vi "CONTROL LIFT ARM.vi"(10 "LIFT ARM refname":string="INTAKE LIFT", 11 "LIFT DRIVE refname":string="INTAKE DRIVE") -> ()   [LabVIEW 2020]
uses:
  <vilib>/Rock Robotics/WPI/ThirdParty/Phoenix-LabVIEW/Motor Controller/Controls/CTRE_Phoenix_MotorControl_ControlMode.ctl
  <vilib>/Rock Robotics/Network Tables/NT Read Boolean.vi
  Robot Global Data.vi
  <vilib>/Rock Robotics/Network Tables/NT Write Boolean.vi
panel:
  out "Sensor Position RETRACT":dbl
  out "TARGET RETRACT":dbl
  out "TARGET EXTEND":dbl
  out "Sensor Position EXTEND":dbl
  in  "degrees overtravel":dbl=5.0 format="%#_13g"
  out "LOOP ITERATION LIMIT?":bool
  out "THRESHOLD?":bool
  out "AND nots":bool[](array[boolean])=[TRUE, FALSE, FALSE, FALSE]
  out "NOT XOR":bool[](array[boolean])=[TRUE, FALSE, FALSE, TRUE]
  out "Not AND":bool[](array[boolean])=[TRUE, TRUE, TRUE, FALSE]
  out "AND?":bool[](array[boolean])=[FALSE, FALSE, FALSE, TRUE]
  in  "POSSIBILITIES":cluster{"EXTEND":bool, "RETRACTED":bool}[](array[cluster])=[{"EXTEND"=FALSE, "RETRACTED"=FALSE}, {"EXTEND"=TRUE, "RETRACTED"=FALSE}, {"EXTEND"=FALSE, "RETRACTED"=TRUE}, {"EXTEND"=TRUE, "RETRACTED"=TRUE}]
  out "IS RETRACTED?":bool
  out "SHOULD BE EXTENDED?":bool
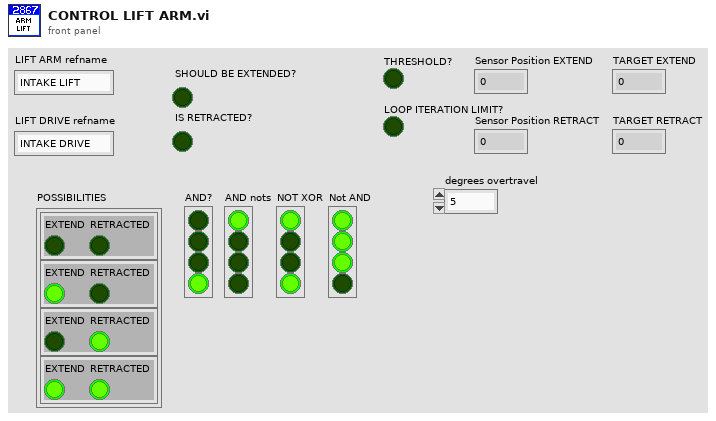
[diagram p1: front panel]
types:
  T1 = cluster{"planetary gear ratio:1":i32, "GEAR TEETH on planetary":i32, "GEAR TEETH on lift arm":i32, "convert motor revs to lift degrees":dbl, "MIN (deg)":dbl, "MAX (deg)":dbl, "roller speed%":dbl, "tip over (deg)":dbl, "lift speed% EXTEND":dbl, "lift speed% RETRACT":dbl}
  T2 = typedef "WPI_MotorControlDeviceRef.ctl" = cluster{"DeviceStatus":errorcluster, "Type":T3, "PWM":cluster{"PWM Channel":T4, "DeadBand":T5}, "CAN":cluster{"Device Number":u8, "SetOutput VI Ref":variant, "GetOutput VI Ref":variant, "Enable VI Ref":variant, "Disable VI Ref":variant, "Data":variant}, "Invert":bool, "DIO PWM":cluster{"PWM \"Enable\" Channel":T4, "DIOChannel":T6, "PWM Rate":dbl}}
  T3 = typedef "WPI_MotorControlType.ctl" = enum16{"PWM", "CAN", "DIO PWM"}
  T4 = typedef "FPGA_DIOPWMChannel.ctl" = enum8{"PWM 0", "PWM 1", "PWM 2", "PWM 3", "PWM 4", "PWM 5", "PWM 6", "PWM 7", "PWM 8", "PWM 9", "PWM MXP 0", "PWM MXP 1", "PWM MXP 2", "PWM MXP 3", "PWM MXP 4", "PWM MXP 5", "PWM MXP 6", "PWM MXP 7", "PWM MXP 8", "PWM MXP 9", "Invalid"}
  T5 = typedef "WPI_PWMDeadband.ctl" = cluster{"Name":string, "maxPositivePwm":i32, "minPositivePwm":i32, "centerPwm":i32, "maxNegativePwm":i32, "minNegativePwm":i32, "angularRange":u16}
  T6 = typedef "FPGA_DIOChannel.ctl" = enum8{"DIO 0", "DIO 1", "DIO 2", "DIO 3", "DIO 4", "DIO 5", "DIO 6", "DIO 7", "DIO 8", "DIO 9", "DIO MXP 0", "DIO MXP 1", "DIO MXP 2", "DIO MXP 3", "DIO MXP 4", "DIO MXP 5", "DIO MXP 6", "DIO MXP 7", "DIO MXP 8", "DIO MXP 9", "DIO MXP 10", "DIO MXP 11", "DIO MXP 12", "DIO MXP 13", "DIO MXP 14", "DIO MXP 15", "SPI Port CS1", "SPI Port CS2", "SPI Port CS3", "SPI Port MISO", "SPI Port MOSI", "Invalid"}
  T7 = typedef "CTRE_Phoenix_MotorControl_ControlMode.ctl" = u16
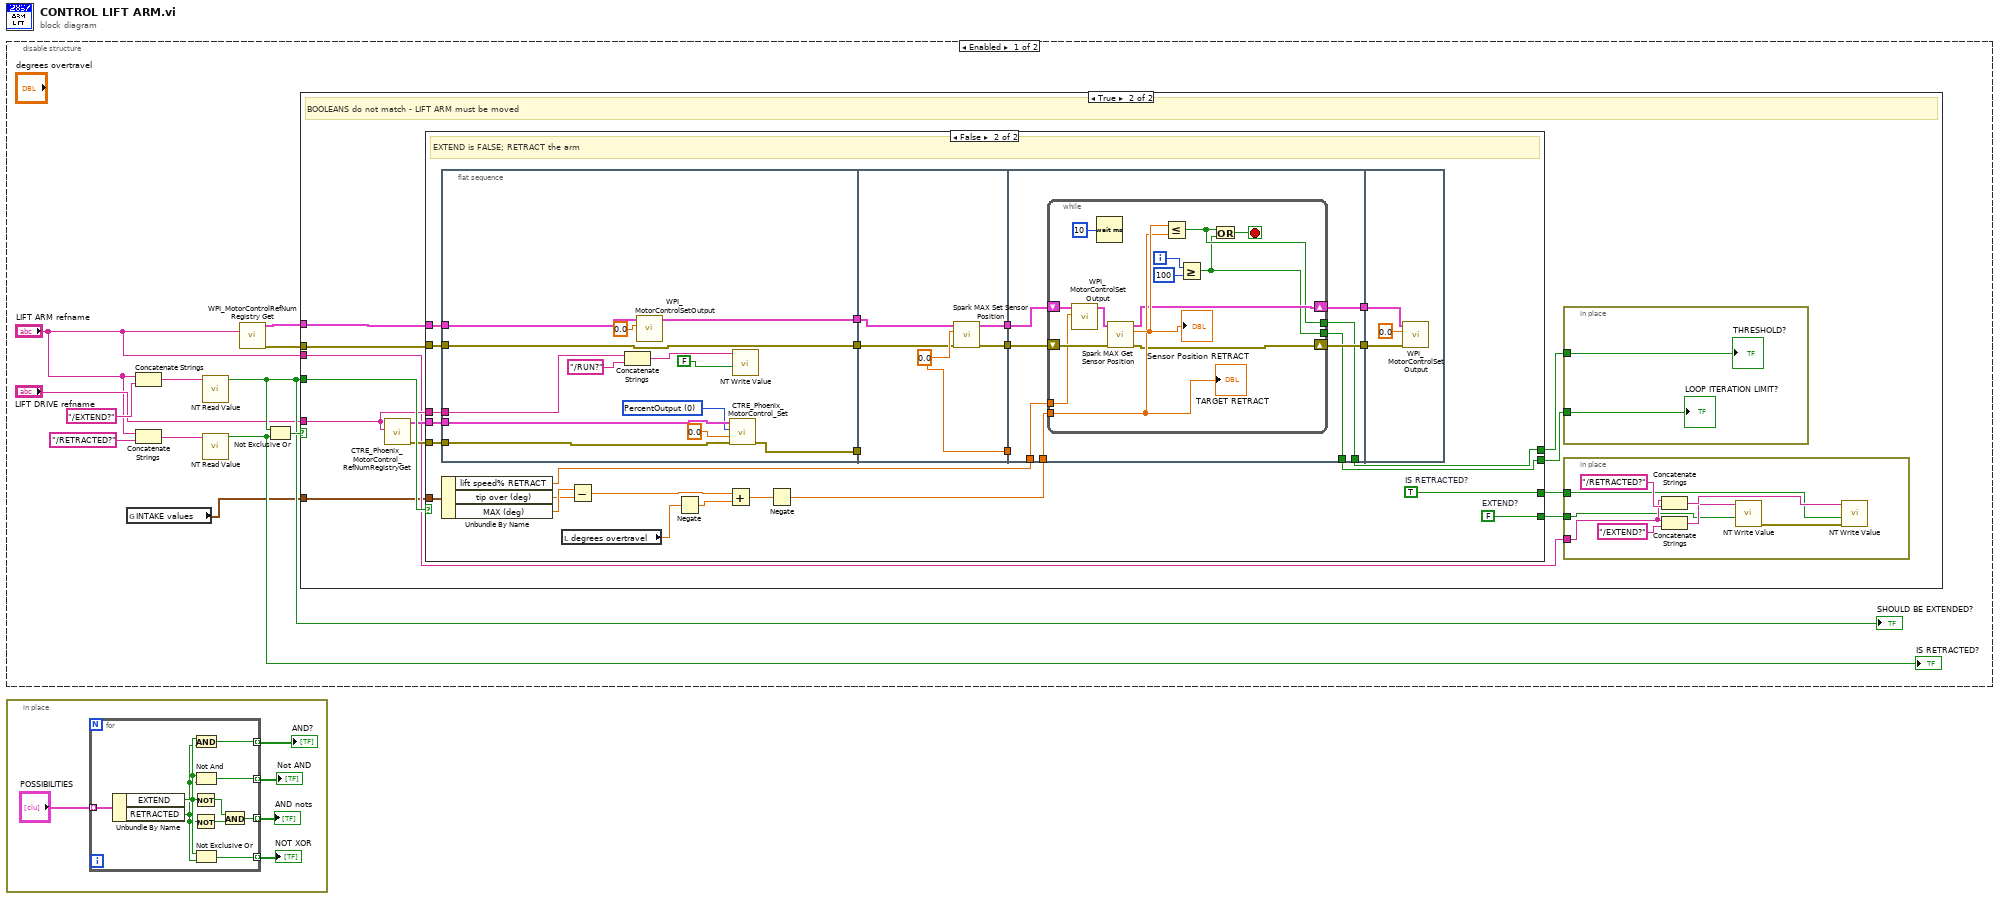
[diagram p0: block diagram]
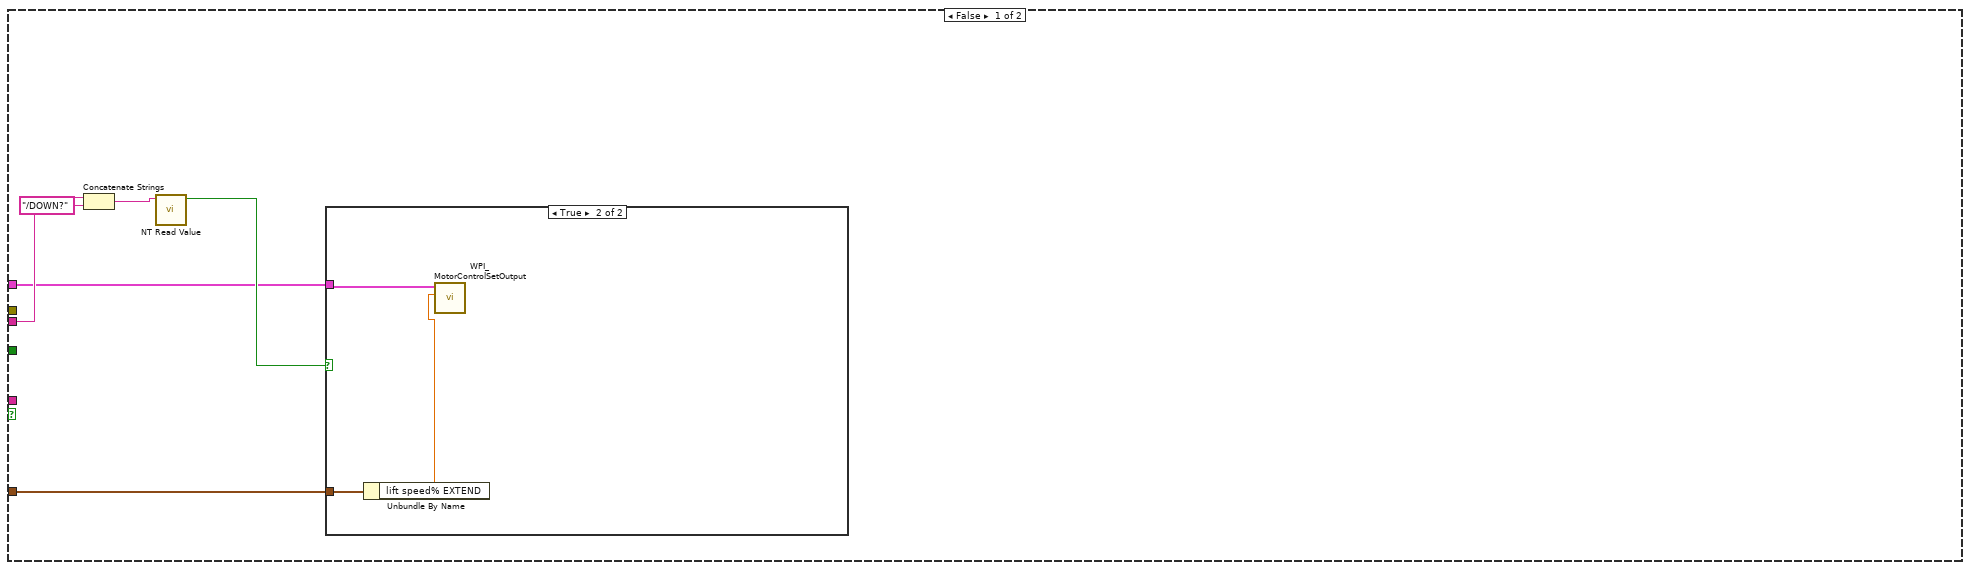
[diagram p2: hidden frame]
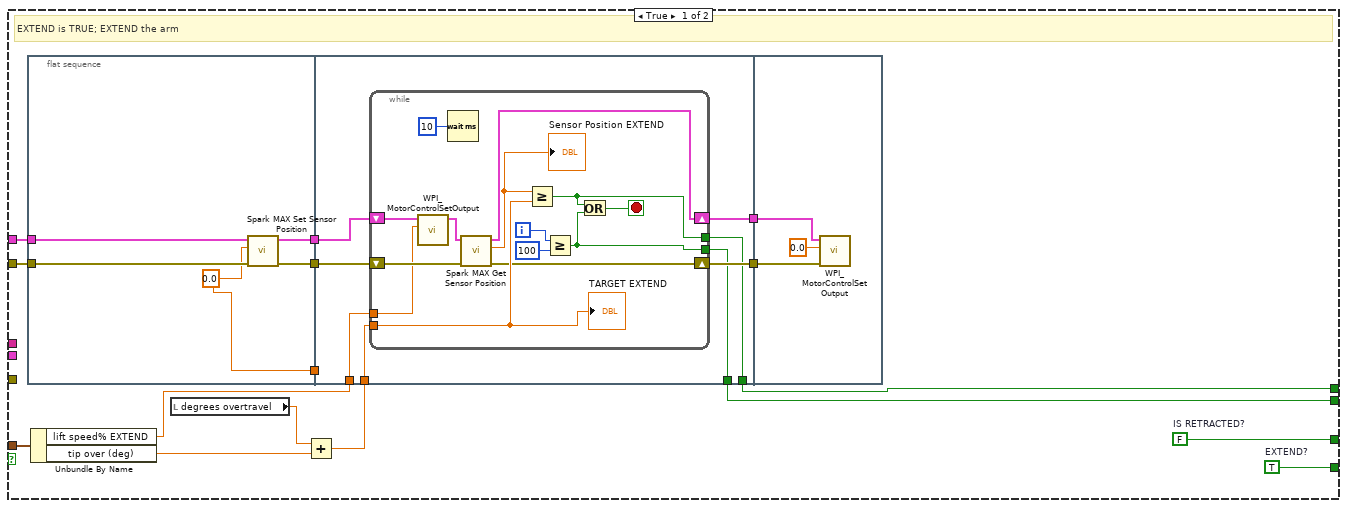
[diagram p4: hidden frame]
diagram:
  n1 = disable-structure shown="Enabled" {
    frame Enabled {
      n2 = global read "Robot Global Data.vi" "INTAKE values"() -> (w1:T1)
      n3 = Concatenate Strings("LIFT ARM refname", "/EXTEND?" ("string")) -> (w5:string)
      n4 = Concatenate Strings("LIFT ARM refname", "/RETRACTED?" ("string")) -> (w10:string)
      n5 = call-poly <vilib>:"NT Read Value.vi"("Name"=w5) -> ("Boolean"=w7:bool)  [unwired: 9 in, 1 out]
      "SHOULD BE EXTENDED?" <- w7
      n6 = call-poly <vilib>:"NT Read Value.vi"("Name"=w10) -> ("Boolean"=w9:bool)  [unwired: 9 in, 1 out]
      "IS RETRACTED?" <- w9
      n7 = call <vilib>:"WPI_MotorControlRefNum Registry Get.vi"("refnum name"="LIFT ARM refname") -> ("error out"=w3:errorcluster, "MotorControlDevRef"=w2:T2)  [unwired: 9 in]
      n8 = Not Exclusive Or(1:w9, 2:w7) -> (0:w8:bool)
      n9 = case shown="True" w8 {
        tunnel: w7 -> [_ w33]
        tunnel: "LIFT DRIVE refname" -> [_ w26]
        tunnel: "LIFT ARM refname" -> [w18 w25]
        tunnel: w3 -> [_ w24]
        tunnel: w2 -> [w14 w23]
        tunnel: w1 -> [w13 w22]
        frame False {
          n10 = Concatenate Strings(w18, "/DOWN?" ("string")) -> (w17:string)
          n11 = call-poly <vilib>:"NT Read Value.vi"("Name"=w17) -> ("Boolean"=w15:bool)  [unwired: 9 in, 1 out]
          n12 = case shown="True" w15 {
            tunnel: w14 -> [_ w20]
            tunnel: w13 -> [_ w21]
            frame False {
            }
            frame True {
              n13 = Unbundle By Name(w21) -> ("lift speed% EXTEND"=w19:dbl)
              n14 = call <vilib>:"WPI_MotorControlSetOutput.vi"("Output"=w19, "MotorControlDevRef"=w20) -> ()  [unwired: 7 in, 3 out]
            }
          }
        }
        frame True {
          # "BOOLEANS do not match - LIFT ARM must be moved"
          n15 = call <vilib>:"CTRE_Phoenix_MotorControl_RefNumRegistryGet.vi"("refnum name"=w26) -> ("error out"=w29:errorcluster, "PhoenixMotorControlDevRef"=w30:T2)  [unwired: 9 in]
          n16 = case shown="False" w33 {
            tunnel: w22 -> [w59 w115]
            tunnel: [w51 w105] -> w32
            tunnel: [w50 w104] -> w31
            tunnel: w24 -> [w48 w103]
            tunnel: w23 -> [w49 w102]
            tunnel: w30 -> [_ w99]
            tunnel: w29 -> [_ w98]
            tunnel: [w47 w96] -> w28
            tunnel: [w46 w95] -> w27
            tunnel: w26 -> [_ w94]
            frame True {
              w46 = FALSE  # IS RETRACTED?
              w47 = TRUE  # EXTEND?
              # "EXTEND is TRUE; EXTEND the arm"
              n17 = flat-sequence {
                tunnel: w49 -> [w64]
                tunnel: [w63] -> w58
                tunnel: [w62] -> w57
                tunnel: w48 -> [w61]
                tunnel: [w60] -> w56
                tunnel: w58 -> [w72]
                tunnel: w57 -> [w71]
                tunnel: w56 -> [_]
                tunnel: w55 -> [w70]
                tunnel: w45 -> [w69]
                tunnel: [w68] -> w53
                tunnel: [w67] -> w52
                tunnel: [w66] -> w51
                tunnel: [w65] -> w50
                tunnel: w53 -> [w89]
                tunnel: w52 -> [w88]
                frame #0 {
                  w60 = 0.0 ("Position")
                  n18 = call <vilib>:"Spark MAX Set Sensor Position.vi"("error in"=w61, "Position"=w60, "MotorControlDeviceRef"=w64) -> ("error out"=w62:errorcluster, "MotorControlDeviceRef"=w63:T2)  [unwired: 7 in]
                }
                frame #1 {
                  n19 = while {
                    shift-right: [w76] -> w67
                    shift-left: w71 -> [w85]
                    shift-right: [w77] -> w68
                    shift-left: w72 -> [w86]
                    tunnel: w70 -> [w75]
                    tunnel: w69 -> [w82]
                    tunnel: [w74] -> w66
                    tunnel: [w73] -> w65
                    i -> [w79]
                    stop <- w80 stop-if-true
                    n20 = call <vilib>:"WPI_MotorControlSetOutput.vi"("Output"=w75, "MotorControlDevRef"=w86) -> ("MotorControlDevRef"=w84:T2)  [unwired: 7 in, 2 out]
                    n21 = Wait (ms)(milliseconds to wait=u32 10) -> ()  [unwired: 1 out]
                    n22 = call <vilib>:"Spark MAX Get Sensor Position.vi"("error in (no error)"=w85, "MotorControlDevRef in"=w84) -> ("error out"=w76:errorcluster, "Sensor Position"=w83:dbl, "MotorControlDevRef out"=w77:T2)  [unwired: 6 in, 1 out]
                    "Sensor Position EXTEND" <- w83
                    n23 = Greater Or Equal?(x=w83, y=w82) -> (x >= y?=w74:bool)
                    n24 = Greater Or Equal?(x=w79, y=100) -> (x >= y?=w73:bool)
                    n25 = Or(x=w74, y=w73) -> (x .or. y?=w80:bool)
                    "TARGET EXTEND" <- w82
                  }
                }
                frame #2 {
                  n26 = call <vilib>:"WPI_MotorControlSetOutput.vi"("error in (no error)"=w88, "Output"=0.0, "MotorControlDevRef"=w89) -> ()  [unwired: 6 in, 3 out]
                }
              }
              n27 = Unbundle By Name(w59) -> ("lift speed% EXTEND"=w55:dbl, "tip over (deg)"=w54:dbl)
              n28 = local read "degrees overtravel"() -> (w44:dbl)
              n29 = Add(x=w44, y=w54) -> (x+y=w45:dbl)
            }
            frame False {
              w95 = TRUE  # IS RETRACTED?
              w96 = FALSE  # EXTEND?
              # "EXTEND is FALSE; RETRACT the arm"
              n30 = flat-sequence {
                tunnel: w102 -> [w127]
                tunnel: w103 -> [w128]
                tunnel: [w128] -> w101
                tunnel: [w122] -> w100
                tunnel: w99 -> [w126]
                tunnel: w98 -> [w125]
                tunnel: [w120] -> w97
                tunnel: w94 -> [w117]
                tunnel: [w133] -> w114
                tunnel: [w132] -> w113
                tunnel: [w131] -> w112
                tunnel: w101 -> [w130]
                tunnel: w100 -> [w129]
                tunnel: w97 -> [_]
                tunnel: w114 -> [w141]
                tunnel: w113 -> [w140]
                tunnel: w112 -> [_]
                tunnel: w111 -> [w139]
                tunnel: w106 -> [w138]
                tunnel: [w137] -> w110
                tunnel: [w136] -> w109
                tunnel: [w135] -> w105
                tunnel: [w134] -> w104
                tunnel: w110 -> [w158]
                tunnel: w109 -> [w157]
                frame #0 {
                  w124 = T7 0 items=["PercentOutput"=0, "Position"=1, "Velocity"=2, "Current"=3, "Follower"=5, "MotionProfile"=6, "MotionMagic"=7, "MotionProfileArc"=10, "Disabled"=15] ("Control Mode")
                  n31 = Concatenate Strings(w117, "/RUN?" ("Name")) -> (w118:string)
                  n32 = call <vilib>:"WPI_MotorControlSetOutput.vi"("Output"=0.0, "MotorControlDevRef"=w127) -> ("MotorControlDevRef"=w122:T2)  [unwired: 7 in, 2 out]
                  n33 = call <vilib>:"CTRE_Phoenix_MotorControl_Set.vi"("error in (no error)"=w125, "Output"=0.0, "Control Mode"=w124, "PhoenixMotorControlDevRef"=w126) -> ("error out"=w120:errorcluster)  [unwired: 6 in, 1 out]
                  n34 = call-poly <vilib>:"NT Write Value.vi"("Boolean"=FALSE, "Name"=w118) -> ()  [unwired: 9 in, 1 out]
                }
                frame #1 {
                  w131 = 0.0 ("Position")
                  n35 = call <vilib>:"Spark MAX Set Sensor Position.vi"("error in"=w130, "Position"=w131, "MotorControlDeviceRef"=w129) -> ("error out"=w132:errorcluster, "MotorControlDeviceRef"=w133:T2)  [unwired: 7 in]
                }
                frame #2 {
                  n36 = while {
                    shift-right: [w145] -> w136
                    shift-left: w140 -> [w154]
                    shift-right: [w146] -> w137
                    shift-left: w141 -> [w155]
                    tunnel: w139 -> [w142]
                    tunnel: w138 -> [w151]
                    tunnel: [w144] -> w135
                    tunnel: [w143] -> w134
                    i -> [w148]
                    stop <- w149 stop-if-true
                    n37 = call <vilib>:"WPI_MotorControlSetOutput.vi"("Output"=w142, "MotorControlDevRef"=w155) -> ("MotorControlDevRef"=w153:T2)  [unwired: 7 in, 2 out]
                    n38 = Wait (ms)(milliseconds to wait=u32 10) -> ()  [unwired: 1 out]
                    n39 = call <vilib>:"Spark MAX Get Sensor Position.vi"("error in (no error)"=w154, "MotorControlDevRef in"=w153) -> ("error out"=w145:errorcluster, "Sensor Position"=w152:dbl, "MotorControlDevRef out"=w146:T2)  [unwired: 6 in, 1 out]
                    "Sensor Position RETRACT" <- w152
                    n40 = Less Or Equal?(x=w152, y=w151) -> (x <= y?=w144:bool)
                    n41 = Greater Or Equal?(x=w148, y=100) -> (x >= y?=w143:bool)
                    n42 = Or(x=w144, y=w143) -> (x .or. y?=w149:bool)
                    "TARGET RETRACT" <- w151
                  }
                }
                frame #3 {
                  n43 = call <vilib>:"WPI_MotorControlSetOutput.vi"("error in (no error)"=w157, "Output"=0.0, "MotorControlDevRef"=w158) -> ()  [unwired: 6 in, 3 out]
                }
              }
              n44 = Unbundle By Name(w115) -> ("lift speed% RETRACT"=w111:dbl, "tip over (deg)"=w107:dbl, "MAX (deg)"=w108:dbl)
              n45 = local read "degrees overtravel"() -> (w91:dbl)
              n46 = Subtract(x=w108, y=w107) -> (x-y=w92:dbl)
              n47 = Negate(x=w91) -> (-x=w90:dbl)
              n48 = Add(x=w92, y=w90) -> (x+y=w93:dbl)
              n49 = Negate(x=w93) -> (-x=w106:dbl)
            }
          }
          n50 = in-place {
            in-place-border: w32 -> [w43]
            in-place-border: w31 -> [w42]
            "THRESHOLD?" <- w43
            "LOOP ITERATION LIMIT?" <- w42
          }
          n51 = in-place {
            in-place-border: w25 -> [w39]
            in-place-border: w28 -> [w36]
            in-place-border: w27 -> [w35]
            n52 = Concatenate Strings(w39, "/RETRACTED?" ("string")) -> (w38:string)
            n53 = Concatenate Strings(w39, "/EXTEND?" ("string")) -> (w37:string)
            n54 = call-poly <vilib>:"NT Write Value.vi"("Boolean"=w36, "Name"=w37) -> ("error out"=w34:errorcluster)  [unwired: 9 in]
            n55 = call-poly <vilib>:"NT Write Value.vi"("error in"=w34, "Boolean"=w35, "Name"=w38) -> ()  [unwired: 8 in, 1 out]
          }
        }
      }
    }
    frame Disabled {
    }
  }
  n56 = in-place {
    n57 = for {
      tunnel: "POSSIBILITIES" -> [w172] mode=indexing
      tunnel: [w169] -> w160 mode=indexing
      tunnel: [w171] -> w161 mode=indexing
      tunnel: [w170] -> w162 mode=indexing
      tunnel: [w164] -> w159 mode=indexing
      n58 = Unbundle By Name(w172) -> ("EXTEND"=w168:bool, "RETRACTED"=w167:bool)
      n59 = Not(x=w168) -> (.not. x?=w166:bool)
      n60 = Not(x=w167) -> (.not. x?=w165:bool)
      n61 = And(x=w168, y=w167) -> (x .and. y?=w170:bool)
      n62 = Not And(1:w167, 2:w168) -> (0:w171:bool)
      n63 = Not Exclusive Or(1:w167, 2:w168) -> (0:w169:bool)
      n64 = And(x=w166, y=w165) -> (x .and. y?=w164:bool)
    }
    "AND?" <- w162
    "Not AND" <- w161
    "NOT XOR" <- w160
    "AND nots" <- w159
  }
